vi "Sequencer Main - Copy.vi"() -> ()   [LabVIEW 2018] (continued)
                              n2084 = Add(1:w4034, 2:w4038) -> (0:w4062:dynamicdata)  [unwired: 1 in, 1 out]
                              n2085 = Multiply(x=w4027, y=w4022) -> (x*y=w4025:dynamicdata)
                              n2086 = Multiply(x=w4065, y=w4022) -> (x*y=w4061:dynamicdata)
                              n2087 = Multiply(x=w4064, y=w4022) -> (x*y=w4060:dynamicdata)
                              n2088 = local read "Measure Ch-A"() -> (w4069:T10)
                              n2089 = Multiply(x=w4030, y=w4022) -> (x*y=w4024:dynamicdata)
                              n2090 = Multiply(x=w4063, y=w4022) -> (x*y=w4059:dynamicdata)
                              n2091 = Multiply(x=w4062, y=w4022) -> (x*y=w4058:dynamicdata)
                              n2092 = Bundle By Name(cluster=w4069, "MAX Vpp"=w4061, "PickToPoick / 2"=w4025, "MIN Vpp"=w4060) -> (w4068:T10)
                              n2093 = local read "Measure Ch-B"() -> (w4066:T9)
                              n2094 = Bundle By Name(cluster=w4066, "MAX Vpp"=w4059, "PickToPick / 2"=w4024, "MIN Vpp"=w4058) -> (w4067:T9)
                              n2095 = local write "Measure Ch-B"(w4067) -> ()
                              n2096 = local write "Measure Ch-A"(w4068) -> ()
                            }
                            frame #2 {
                              # "GoTo Test-nmb"
                              # "ReTest Cyckles"
                              # "Select Channel & Set Retest Parametrs in FALSE Case"
                              n2097 = Index Array(array=w4082, index #1=0 ("index"), index #2=1 ("index"), index #3=2 ("index")) -> (element #1=w4086:string, element #2=w4087:string, element #3=w4088:string)
                              n2098 = global read "Global Variable.vi" "Retest Cnt"() -> (w4081:i16)
                              n2099 = local read "Debugging"() -> (w4079:bool)
                              n2100 = To Upper Case(1:w4086) -> (0:w4078:string)
                              n2101 = call "Convert from Dynamic Data8"("Dynamic Data Type"=w4074) -> ("Scalar"=w4070:dbl)  [unwired: 3 in]
                              n2102 = call "Convert from Dynamic Data6"("Dynamic Data Type"=w4073) -> ("Scalar"=w4071:dbl)  [unwired: 3 in]
                              n2103 = Decimal String To Number(string=w4088) -> (number=w4075:i32)  [unwired: 2 in, 1 out]
                              n2104 = Decimal String To Number(string=w4087) -> (number=w4077:i32)  [unwired: 2 in, 1 out]
                              n2105 = Equal?(x=w4081, y=i16 0) -> (x = y?=w4076:bool)
                              n2106 = case shown="False" w4079 {
                                tunnel: w4078 -> [w4093 _]
                                tunnel: w4076 -> [w4090 _]
                                tunnel: w4075 -> [w4092 _]
                                tunnel: w4077 -> [w4091 _]
                                frame False {
                                n2107 = case shown="\"FALSE\"" w4093 {
                                tunnel: w4090 -> [_ w4097]
                                tunnel: w4092 -> [_ w4094]
                                tunnel: w4091 -> [_ w4095]
                                frame "Idle", Default {
                                }
                                frame "FALSE" {
                                n2108 = global write "Global Variable.vi" "Retest Step Nmb"(w4095) -> ()
                                n2109 = global write "Global Variable.vi" "Retest Nmb"(w4094) -> ()
                                n2110 = case shown="True" w4097 {
                                tunnel: w4094 -> [_ w4101]
                                tunnel: w4095 -> [_ _]
                                frame False {
                                n2111 = global read "Global Variable.vi" "Retest Cnt"() -> (w4099:i16)
                                n2112 = Decrement(x=w4099) -> (x-1=w4098:i16)
                                n2113 = global write "Global Variable.vi" "Retest Cnt"(w4098) -> ()
                                }
                                frame True {
                                # "if(Retest-OFF & Cnt=0)"
                                n2114 = Decrement(x=w4101) -> (x-1=w4100:i32)
                                n2115 = global write "Global Variable.vi" "Retest Cnt"(w4100) -> ()
                                }
                                }
                                n2116 = global write "Global Variable.vi" "Retest ON"(TRUE ("Retest ON")) -> ()
                                }
                                }
                                }
                                frame True {
                                }
                              }
                              n2117 = case shown="\"A\", Default" w4089 {
                                tunnel: [w4102 w4103] -> w4072
                                tunnel: w4071 -> [_ w4103]
                                tunnel: w4070 -> [w4102 _]
                                frame "A", Default {
                                }
                                frame "B" {
                                }
                              }
                            }
                            frame #3 {
                              n2118 = local read "Delay"() -> (w4104:u16)
                              n2119 = Multiply(x=w4104, y=u32 1000 ("milliseconds to wait")) -> (x*y=w4106:u32)
                              n2120 = Wait (ms)(milliseconds to wait=w4106) -> ()  [unwired: 1 out]
                            }
                          }
                          n2121 = in-place {
                            in-place-border: w3964 -> [w3987]
                            in-place-border: w3965 -> [w3981]
                            in-place-border: w3966 -> [w3980]
                            in-place-border: [w3988] -> w3962
                            in-place-border: [w3986] -> w3961
                            # "Step Result Msg"
                            # "Step TEST Result"
                            n2122 = In Range and Coerce(upper limit=w3981, x=w3987, lower limit=w3980) -> (In Range?=w3984:bool)  [unwired: 1 out]
                            n2123 = And(x=w3984, y=TRUE) -> (x .and. y?=w3983:bool)
                            n2124 = case shown="False" w3983 {
                              tunnel: [enum16{"Idle", "PASS", "FALSE"}."FALSE" ("Step Test Result") enum16{"Idle", "PASS", "FALSE"}."PASS" ("Step Test Result")] -> w3988
                              frame False {
                              }
                              frame True {
                              }
                            }
                            n2125 = Format Into String(format string="%.1f (V)", w3987) -> (resulting string=w3986:string)  [unwired: 2 in, 1 out]
                          }
                        }
                        frame 53 {
                          # "Read Only POSITIVE or NEGATIVE Values"
                          # "Read Arrays Of DATA"
                          # "Lover Lim"
                          # "Upper Lim"
                          # "PicoScope Case\nPositive / Negative"
                          # "PicoScope Case"
                          n2126 = Unbundle By Name(w4131) -> ("Parameters"=w4125:string, "Test Values.Upper Limit"=w4129:dbl, "Test Values.Lower Limit"=w4128:dbl, "Test Values.Numeric Value"=w4130:dbl)
                          n2127 = property on="Tab Control Msg" class="TabCtl (strict)"("Value"=T21."Scope" ("Tab Control Msg")) -> (error out=w4127:errorcluster)  [unwired: 2 in, 1 out]
                          n2128 = flat-sequence {
                            tunnel: w4130 -> [w4163]
                            tunnel: w4129 -> [w4156]
                            tunnel: w4128 -> [w4155]
                            tunnel: w4127 -> [_]
                            tunnel: [w4156] -> w4115
                            tunnel: [w4155] -> w4116
                            tunnel: w4125 -> [w4154]
                            tunnel: [w4152] -> w4120
                            tunnel: [w4149] -> w4117
                            tunnel: [w4146] -> w4109
                            tunnel: [w4194] -> w4124
                            tunnel: [w4193] -> w4123
                            tunnel: [w4192] -> w4122
                            tunnel: [w4191] -> w4121
                            tunnel: w4120 -> [w4180]
                            tunnel: [w4180] -> w4119
                            tunnel: [w4179] -> w4118
                            tunnel: w4117 -> [w4179]
                            tunnel: [w4177] -> w4110
                            tunnel: w4109 -> [w4177]
                            tunnel: [w4234] -> w4114
                            tunnel: [w4236] -> w4113
                            tunnel: w4124 -> [w4235]
                            tunnel: w4123 -> [w4233]
                            tunnel: w4122 -> [w4232]
                            tunnel: w4121 -> [w4231]
                            tunnel: w4119 -> [w4230]
                            tunnel: w4118 -> [w4223]
                            tunnel: w4110 -> [w4215]
                            tunnel: [w4214] -> w4108
                            frame #0 {
                              n2129 = while {
                                shift-right: [w4174] -> _
                                shift-left: w4154 -> [w4175]
                                tunnel: [w4171] -> w4153 mode=indexing
                                stop <- w4173 stop-if-true
                                # "Get Array of Parametrs"
                                n2130 = Match Pattern(string=w4175, regular expression=">") -> (before substring=w4171:string, after substring=w4174:string, offset past match=w4172:i32)  [unwired: 1 in, 1 out]
                                n2131 = Less Than 0?(x=w4172) -> (x < 0?=w4173:bool)
                              }
                              n2132 = Multiply(x=w4155, y=-0.2) -> (x*y=w4158:dbl)
                              n2133 = Bundle("Lower Limit"=w4155, "Upper Limit"=w4156, "Numeric Value"=w4163) -> (w4164:T36)  [unwired: 1 in]
                              n2134 = Multiply(x=w4156, y=0.2) -> (x*y=w4160:dbl)
                              n2135 = Add(x=w4158, y=w4155) -> (x+y=w4157:dbl)
                              n2136 = property on="Limits" class="Slide (strict)"("Value"=w4164) -> ()  [unwired: 2 in, 2 out]
                              n2137 = Add(x=w4160, y=w4156) -> (x+y=w4159:dbl)
                              n2138 = property on="Limits" class="Slide (strict)"("Scale.Maximum"=w4159, "Scale.Minimum"=w4157) -> ()  [unwired: 2 in, 2 out]
                              n2139 = Index Array(array=w4153, index #1=0 ("index"), index #2=1 ("index"), index #3=2 ("index")) -> (element #1=w4152:string, element #2=w4146:string, element #3=w4147:string)
                              n2140 = while {
                                shift-right: [w4168] -> _
                                shift-left: w4147 -> [w4169]
                                tunnel: [w4165] -> w4149 mode=indexing
                                stop <- w4167 stop-if-true
                                # "Get Array of Sub Parametrs"
                                n2141 = Match Pattern(string=w4169, regular expression=":") -> (before substring=w4165:string, after substring=w4168:string, offset past match=w4166:i32)  [unwired: 1 in, 1 out]
                                n2142 = Less Than 0?(x=w4166) -> (x < 0?=w4167:bool)
                              }
                            }
                            frame #1 {
                              w4184 = 700 ("index")
                              w4178 = 290.0
                              # "302"
                              # "Devider compensite"
                              # "remove first\nxx element (noise)"
                              # "Ch-B Negative Vmin"
                              # "Ch-B Positive Vmax"
                              # "Ch-A Negative Vmin"
                              # "Ch-A Positive Vmax"
                              # "Res Devider Compens\n100K / 10K"
                              # "Calculate Values"
                              n2143 = local read "Channel A"() -> (w4213:cluster{i32, dbl, dbl[]})
                              n2144 = local read "Channel B"() -> (w4208:cluster{i32, dbl, dbl[]})
                              n2145 = Unbundle(w4213) -> (w4181:dbl[])  [unwired: 2 out]
                              n2146 = Unbundle(w4208) -> (w4186:dbl[])  [unwired: 2 out]
                              n2147 = Array Size(array=w4181) -> (size(s)=w4189:i32)
                              n2148 = Array Size(array=w4186) -> (size(s)=w4185:i32)
                              n2149 = Subtract(x=w4189, y=w4184) -> (x-y=w4188:i32)
                              n2150 = Array Subset(array=w4181, index=w4184, length=w4188) -> (w4190:dbl[])
                              n2151 = Subtract(x=w4185, y=w4184) -> (x-y=w4183:i32)
                              n2152 = Array Subset(array=w4186, index=w4184, length=w4183) -> (w4187:dbl[])
                              n2153 = call-poly <vilib>:"Basic Averaged DC-RMS.vi"("signal in"=w4190) -> ("RMS value"=w4202:dbl, "DC value"=w4182:dbl)  [unwired: 7 in, 2 out]
                              n2154 = Array Max & Min(array=w4190) -> (max value=w4210:dbl, min value=w4209:dbl)  [unwired: 2 out]
                              n2155 = call-poly <vilib>:"Basic Averaged DC-RMS.vi"("signal in"=w4187) -> ("RMS value"=w4198:dbl, "DC value"=w4207:dbl)  [unwired: 7 in, 2 out]
                              n2156 = Array Max & Min(array=w4187) -> (max value=w4205:dbl, min value=w4206:dbl)  [unwired: 2 out]
                              n2157 = Subtract(x=w4210, y=w4182) -> (x-y=w4201:dbl)
                              n2158 = Add(x=w4209, y=w4182) -> (x+y=w4200:dbl)
                              n2159 = Subtract(x=w4205, y=w4207) -> (x-y=w4196:dbl)
                              n2160 = Add(x=w4206, y=w4207) -> (x+y=w4195:dbl)
                              n2161 = Multiply(x=w4202, y=w4178) -> (x*y=w4199:dbl)
                              n2162 = Multiply(x=w4201, y=w4178) -> (x*y=w4194:dbl)
                              n2163 = Multiply(x=w4200, y=w4178) -> (x*y=w4193:dbl)
                              n2164 = Multiply(x=w4198, y=w4178) -> (x*y=w4197:dbl)
                              n2165 = Multiply(x=w4196, y=w4178) -> (x*y=w4192:dbl)
                              n2166 = Multiply(x=w4195, y=w4178) -> (x*y=w4191:dbl)
                              n2167 = local read "Measure Ch-A"() -> (w4212:T10)
                              n2168 = Bundle By Name(cluster=w4212, "MAX Vpp"=w4194, "PickToPoick / 2"=w4199, "MIN Vpp"=w4193) -> (w4211:T10)
                              n2169 = local read "Measure Ch-B"() -> (w4203:T9)
                              n2170 = local write "Measure Ch-A"(w4211) -> ()
                              n2171 = Bundle By Name(cluster=w4203, "MAX Vpp"=w4192, "PickToPick / 2"=w4197, "MIN Vpp"=w4191) -> (w4204:T9)
                              n2172 = local write "Measure Ch-B"(w4204) -> ()
                            }
                            frame #2 {
                              # "Negative"
                              # "Positive"
                              # "GoTo Test-nmb"
                              # "ReTest Cyckles"
                              # "Select Channel & Set Retest Parametrs in FALSE Case"
                              n2173 = Index Array(array=w4223, index #1=0 ("index"), index #2=1 ("index"), index #3=2 ("index")) -> (element #1=w4227:string, element #2=w4228:string, element #3=w4229:string)
                              n2174 = global read "Global Variable.vi" "Retest Cnt"() -> (w4222:i16)
                              n2175 = local read "Debugging"() -> (w4220:bool)
                              n2176 = To Upper Case(1:w4227) -> (0:w4219:string)
                              n2177 = Decimal String To Number(string=w4229) -> (number=w4216:i32)  [unwired: 2 in, 1 out]
                              n2178 = Decimal String To Number(string=w4228) -> (number=w4218:i32)  [unwired: 2 in, 1 out]
                              n2179 = Equal?(x=w4222, y=i16 0) -> (x = y?=w4217:bool)
                              n2180 = case shown="False" w4220 {
                                tunnel: w4219 -> [w4240 _]
                                tunnel: w4217 -> [w4237 _]
                                tunnel: w4216 -> [w4239 _]
                                tunnel: w4218 -> [w4238 _]
                                frame False {
                                n2181 = case shown="\"FALSE\"" w4240 {
                                tunnel: w4237 -> [_ w4244]
                                tunnel: w4239 -> [_ w4241]
                                tunnel: w4238 -> [_ w4242]
                                frame "Idle", Default {
                                }
                                frame "FALSE" {
                                n2182 = global write "Global Variable.vi" "Retest Step Nmb"(w4242) -> ()
                                n2183 = global write "Global Variable.vi" "Retest Nmb"(w4241) -> ()
                                n2184 = case shown="True" w4244 {
                                tunnel: w4241 -> [_ w4248]
                                tunnel: w4242 -> [_ _]
                                frame False {
                                n2185 = global read "Global Variable.vi" "Retest Cnt"() -> (w4246:i16)
                                n2186 = Decrement(x=w4246) -> (x-1=w4245:i16)
                                n2187 = global write "Global Variable.vi" "Retest Cnt"(w4245) -> ()
                                }
                                frame True {
                                # "if(Retest-OFF & Cnt=0)"
                                n2188 = Decrement(x=w4248) -> (x-1=w4247:i32)
                                n2189 = global write "Global Variable.vi" "Retest Cnt"(w4247) -> ()
                                }
                                }
                                n2190 = global write "Global Variable.vi" "Retest ON"(TRUE ("Retest ON")) -> ()
                                }
                                }
                                }
                                frame True {
                                }
                              }
                              n2191 = case shown="\"A\", Default" w4230 {
                                tunnel: [w4250 w4252] -> w4236
                                tunnel: w4235 -> [w4250 _]
                                tunnel: [w4249 w4251] -> w4234
                                tunnel: w4233 -> [w4249 _]
                                tunnel: w4232 -> [_ w4252]
                                tunnel: w4231 -> [_ w4251]
                                frame "A", Default {
                                }
                                frame "B" {
                                }
                              }
                              n2192 = To Lower Case(string=w4215) -> (all lower case string=w4214:string)
                            }
                          }
                          n2193 = in-place {
                            in-place-border: w4113 -> [w4134]
                            in-place-border: w4114 -> [w4133]
                            in-place-border: w4115 -> [w4137]
                            in-place-border: w4116 -> [w4136]
                            in-place-border: [w4141] -> w4112
                            in-place-border: [w4140] -> w4111
                            in-place-border: w4108 -> [w4135]
                            # "Upper Limit Check"
                            # "Step Result Msg"
                            # "Step TEST Result"
                            n2194 = case shown="\"positive\", Default" w4135 {
                              tunnel: w4134 -> [_ w4143]
                              tunnel: w4133 -> [w4142 _]
                              tunnel: [w4142 w4143] -> w4132
                              frame "negative" {
                              }
                              frame "positive", Default {
                              }
                            }
                            n2195 = Format Into String(format string="%.1f (VAC )", w4132) -> (resulting string=w4140:string)  [unwired: 2 in, 1 out]
                            n2196 = In Range and Coerce(upper limit=w4137, x=w4132, lower limit=w4136) -> (In Range?=w4138:bool)  [unwired: 1 out]
                            n2197 = case shown="False" w4138 {
                              tunnel: [enum16{"Idle", "PASS", "FALSE"}."FALSE" ("Step Test Result") enum16{"Idle", "PASS", "FALSE"}."PASS" ("Step Test Result")] -> w4141
                              frame False {
                              }
                              frame True {
                              }
                            }
                          }
                        }
                        frame 54 {
                          # "PicoScope\n     Case\nLower Limit"
                          # "Read Arrays Of DATA"
                          # "Lover Lim"
                          # "Upper Lim"
                          # "PicoScope Case"
                          n2198 = Unbundle By Name(w4273) -> ("Parameters"=w4265:string, "Test Values.Upper Limit"=w4271:dbl, "Test Values.Lower Limit"=w4270:dbl, "Test Values.Numeric Value"=w4272:dbl)
                          n2199 = property on="Tab Control Msg" class="TabCtl (strict)"("Value"=T21."Scope" ("Tab Control Msg")) -> (error out=w4269:errorcluster)  [unwired: 2 in, 1 out]
                          n2200 = flat-sequence {
                            tunnel: w4272 -> [w4298]
                            tunnel: w4271 -> [w4291]
                            tunnel: w4270 -> [w4290]
                            tunnel: w4269 -> [_]
                            tunnel: [w4291] -> w4255
                            tunnel: [w4290] -> w4256
                            tunnel: w4265 -> [w4289]
                            tunnel: [w4287] -> w4260
                            tunnel: [w4283] -> w4257
                            tunnel: [w4328] -> w4264
                            tunnel: [w4327] -> w4263
                            tunnel: [w4326] -> w4262
                            tunnel: [w4325] -> w4261
                            tunnel: w4260 -> [w4314]
                            tunnel: [w4314] -> w4259
                            tunnel: [w4313] -> w4258
                            tunnel: w4257 -> [w4313]
                            tunnel: [w4366] -> w4254
                            tunnel: [w4368] -> w4253
                            tunnel: w4264 -> [w4367]
                            tunnel: w4263 -> [w4365]
                            tunnel: w4262 -> [w4364]
                            tunnel: w4261 -> [w4363]
                            tunnel: w4259 -> [w4362]
                            tunnel: w4258 -> [w4355]
                            frame #0 {
                              n2201 = while {
                                shift-right: [w4309] -> _
                                shift-left: w4289 -> [w4310]
                                tunnel: [w4306] -> w4288 mode=indexing
                                stop <- w4308 stop-if-true
                                # "Get Array of Parametrs"
                                n2202 = Match Pattern(string=w4310, regular expression=">") -> (before substring=w4306:string, after substring=w4309:string, offset past match=w4307:i32)  [unwired: 1 in, 1 out]
                                n2203 = Less Than 0?(x=w4307) -> (x < 0?=w4308:bool)
                              }
                              n2204 = Multiply(x=w4290, y=-0.2) -> (x*y=w4293:dbl)
                              n2205 = Bundle("Lower Limit"=w4290, "Upper Limit"=w4291, "Numeric Value"=w4298) -> (w4299:T36)  [unwired: 1 in]
                              n2206 = Multiply(x=w4291, y=0.2) -> (x*y=w4295:dbl)
                              n2207 = Add(x=w4293, y=w4290) -> (x+y=w4292:dbl)
                              n2208 = property on="Limits" class="Slide (strict)"("Value"=w4299) -> ()  [unwired: 2 in, 2 out]
                              n2209 = Add(x=w4295, y=w4291) -> (x+y=w4294:dbl)
                              n2210 = property on="Limits" class="Slide (strict)"("Scale.Maximum"=w4294, "Scale.Minimum"=w4292) -> ()  [unwired: 2 in, 2 out]
                              n2211 = Index Array(array=w4288, index #1=0 ("index"), index #2=1 ("index")) -> (element #1=w4287:string, element #2=w4284:string)
                              n2212 = while {
                                shift-right: [w4303] -> _
                                shift-left: w4284 -> [w4304]
                                tunnel: [w4300] -> w4283 mode=indexing
                                stop <- w4302 stop-if-true
                                # "Get Array of Sub Parametrs"
                                n2213 = Match Pattern(string=w4304, regular expression=":") -> (before substring=w4300:string, after substring=w4303:string, offset past match=w4301:i32)  [unwired: 1 in, 1 out]
                                n2214 = Less Than 0?(x=w4301) -> (x < 0?=w4302:bool)
                              }
                            }
                            frame #1 {
                              w4318 = 700 ("index")
                              w4312 = 290.0
                              # "302"
                              # "Devider compensite"
                              # "remove first\nxx element (noise)"
                              # "Ch-B Negative Vmin"
                              # "Ch-B Positive Vmax"
                              # "Ch-A Negative Vmin"
                              # "Ch-A Positive Vmax"
                              # "Res Devider Compens\n100K / 10K"
                              # "Calculate Values"
                              n2215 = local read "Channel A"() -> (w4347:cluster{i32, dbl, dbl[]})
                              n2216 = local read "Channel B"() -> (w4342:cluster{i32, dbl, dbl[]})
                              n2217 = Unbundle(w4347) -> (w4315:dbl[])  [unwired: 2 out]
                              n2218 = Unbundle(w4342) -> (w4320:dbl[])  [unwired: 2 out]
                              n2219 = Array Size(array=w4315) -> (size(s)=w4323:i32)
                              n2220 = Array Size(array=w4320) -> (size(s)=w4319:i32)
                              n2221 = Subtract(x=w4323, y=w4318) -> (x-y=w4322:i32)
                              n2222 = Array Subset(array=w4315, index=w4318, length=w4322) -> (w4324:dbl[])
                              n2223 = Subtract(x=w4319, y=w4318) -> (x-y=w4317:i32)
                              n2224 = Array Subset(array=w4320, index=w4318, length=w4317) -> (w4321:dbl[])
                              n2225 = call-poly <vilib>:"Basic Averaged DC-RMS.vi"("signal in"=w4324) -> ("RMS value"=w4336:dbl, "DC value"=w4316:dbl)  [unwired: 7 in, 2 out]
                              n2226 = Array Max & Min(array=w4324) -> (max value=w4344:dbl, min value=w4343:dbl)  [unwired: 2 out]
                              n2227 = call-poly <vilib>:"Basic Averaged DC-RMS.vi"("signal in"=w4321) -> ("RMS value"=w4332:dbl, "DC value"=w4341:dbl)  [unwired: 7 in, 2 out]
                              n2228 = Array Max & Min(array=w4321) -> (max value=w4339:dbl, min value=w4340:dbl)  [unwired: 2 out]
                              n2229 = Subtract(x=w4344, y=w4316) -> (x-y=w4335:dbl)
                              n2230 = Add(x=w4343, y=w4316) -> (x+y=w4334:dbl)
                              n2231 = Subtract(x=w4339, y=w4341) -> (x-y=w4330:dbl)
                              n2232 = Add(x=w4340, y=w4341) -> (x+y=w4329:dbl)
                              n2233 = Multiply(x=w4336, y=w4312) -> (x*y=w4333:dbl)
                              n2234 = Multiply(x=w4335, y=w4312) -> (x*y=w4328:dbl)
                              n2235 = Multiply(x=w4334, y=w4312) -> (x*y=w4327:dbl)
                              n2236 = Multiply(x=w4332, y=w4312) -> (x*y=w4331:dbl)
                              n2237 = Multiply(x=w4330, y=w4312) -> (x*y=w4326:dbl)
                              n2238 = Multiply(x=w4329, y=w4312) -> (x*y=w4325:dbl)
                              n2239 = local read "Measure Ch-A"() -> (w4346:T10)
                              n2240 = Bundle By Name(cluster=w4346, "MAX Vpp"=w4328, "PickToPoick / 2"=w4333, "MIN Vpp"=w4327) -> (w4345:T10)
                              n2241 = local read "Measure Ch-B"() -> (w4337:T9)
                              n2242 = local write "Measure Ch-A"(w4345) -> ()
                              n2243 = Bundle By Name(cluster=w4337, "MAX Vpp"=w4326, "PickToPick / 2"=w4331, "MIN Vpp"=w4325) -> (w4338:T9)
                              n2244 = local write "Measure Ch-B"(w4338) -> ()
                            }
                            frame #2 {
                              # "GoTo Test-nmb"
                              # "ReTest Cyckles"
                              # "Select Channel & Set Retest Parametrs in FALSE Case"
                              n2245 = case shown="\"B\"" w4362 {
                                tunnel: [w4382 w4384] -> w4368
                                tunnel: w4367 -> [w4382 _]
                                tunnel: [w4381 w4383] -> w4366
                                tunnel: w4365 -> [w4381 _]
                                tunnel: w4364 -> [_ w4384]
                                tunnel: w4363 -> [_ w4383]
                                frame "A", Default {
                                }
                                frame "B" {
                                }
                              }
                              n2246 = Index Array(array=w4355, index #1=0 ("index"), index #2=1 ("index"), index #3=2 ("index")) -> (element #1=w4359:string, element #2=w4360:string, element #3=w4361:string)
                              n2247 = global read "Global Variable.vi" "Retest Cnt"() -> (w4354:i16)
                              n2248 = local read "Debugging"() -> (w4352:bool)
                              n2249 = To Upper Case(1:w4359) -> (0:w4351:string)
                              n2250 = Decimal String To Number(string=w4361) -> (number=w4348:i32)  [unwired: 2 in, 1 out]
                              n2251 = Decimal String To Number(string=w4360) -> (number=w4350:i32)  [unwired: 2 in, 1 out]
                              n2252 = Equal?(x=w4354, y=i16 0) -> (x = y?=w4349:bool)
                              n2253 = case shown="False" w4352 {
                                tunnel: w4351 -> [w4372 _]
                                tunnel: w4349 -> [w4369 _]
                                tunnel: w4348 -> [w4371 _]
                                tunnel: w4350 -> [w4370 _]
                                frame False {
                                n2254 = case shown="\"FALSE\"" w4372 {
                                tunnel: w4369 -> [_ w4376]
                                tunnel: w4371 -> [_ w4373]
                                tunnel: w4370 -> [_ w4374]
                                frame "Idle", Default {
                                }
                                frame "FALSE" {
                                n2255 = global write "Global Variable.vi" "Retest Step Nmb"(w4374) -> ()
                                n2256 = global write "Global Variable.vi" "Retest Nmb"(w4373) -> ()
                                n2257 = case shown="True" w4376 {
                                tunnel: w4373 -> [_ w4380]
                                tunnel: w4374 -> [_ _]
                                frame False {
                                n2258 = global read "Global Variable.vi" "Retest Cnt"() -> (w4378:i16)
                                n2259 = Decrement(x=w4378) -> (x-1=w4377:i16)
                                n2260 = global write "Global Variable.vi" "Retest Cnt"(w4377) -> ()
                                }
                                frame True {
                                # "if(Retest-OFF & Cnt=0)"
                                n2261 = Decrement(x=w4380) -> (x-1=w4379:i32)
                                n2262 = global write "Global Variable.vi" "Retest Cnt"(w4379) -> ()
                                }
                                }
                                n2263 = global write "Global Variable.vi" "Retest ON"(TRUE ("Retest ON")) -> ()
                                }
                                }
                                }
                                frame True {
                                }
                              }
                            }
                          }
                          n2264 = in-place {
                            in-place-border: w4253 -> [_]
                            in-place-border: w4254 -> [w4277]
                            in-place-border: w4255 -> [w4275]
                            in-place-border: w4256 -> [w4274]
                            in-place-border: [w4280] -> w4267
                            in-place-border: [w4279] -> w4266
                            # "Step Result Msg"
                            # "Step TEST Result"
                            n2265 = In Range and Coerce(upper limit=w4275, x=w4277, lower limit=w4274) -> (In Range?=w4276:bool)  [unwired: 1 out]
                            n2266 = case shown="False" w4276 {
                              tunnel: [enum16{"Idle", "PASS", "FALSE"}."FALSE" ("Step Test Result") enum16{"Idle", "PASS", "FALSE"}."PASS" ("Step Test Result")] -> w4280
                              frame False {
                              }
                              frame True {
                              }
                            }
                            n2267 = Format Into String(format string="%.1f (VAC)", w4277) -> (resulting string=w4279:string)  [unwired: 2 in, 1 out]
                          }
                        }
                        frame 55 {
                          # "PicoScope\n     Case\nLower Limit"
                          # "Read Arrays Of DATA"
                          # "PicoScope AWG"
                          n2268 = Unbundle By Name(w4402) -> ("Parameters"=w4396:string, "Test Values.Upper Limit"=w4400:dbl, "Test Values.Lower Limit"=w4399:dbl, "Test Values.Numeric Value"=w4401:dbl)
                          n2269 = property on="Tab Control Msg" class="TabCtl (strict)"("Value"=T21."Settings" ("Tab Control Msg")) -> (error out=w4398:errorcluster)  [unwired: 2 in, 1 out]
                          n2270 = flat-sequence {
                            tunnel: w4401 -> [w4426]
                            tunnel: w4400 -> [w4419]
                            tunnel: w4399 -> [w4418]
                            tunnel: w4398 -> [_]
                            tunnel: [w4419] -> _
                            tunnel: [w4418] -> _
                            tunnel: w4396 -> [w4417]
                            tunnel: [w4415] -> w4395
                            tunnel: [w4409] -> w4392
                            tunnel: [w4408] -> w4391
                            tunnel: [w4407] -> w4390
                            tunnel: [w4406] -> w4389
                            tunnel: [w4405] -> w4388
                            tunnel: w4395 -> [w4454]
                            tunnel: w4392 -> [w4453]
                            tunnel: w4391 -> [w4452]
                            tunnel: w4390 -> [w4451]
                            tunnel: w4389 -> [w4450]
                            tunnel: w4388 -> [w4449]
                            tunnel: [w4447] -> w4387
                            frame #0 {
                              n2271 = while {
                                shift-right: [w4433] -> _
                                shift-left: w4417 -> [w4434]
                                tunnel: [w4429] -> w4416 mode=indexing
                                tunnel: [w4428] -> w4405
                                i -> [w4428]
                                stop <- w4432 stop-if-true
                                # "Get Array of Parametrs"
                                n2272 = Match Pattern(string=w4434, regular expression=">") -> (before substring=w4430:string, after substring=w4433:string, offset past match=w4431:i32)  [unwired: 1 in, 1 out]
                                n2273 = Less Than 0?(x=w4431) -> (x < 0?=w4432:bool)
                                n2274 = To Lower Case(string=w4430) -> (all lower case string=w4429:string)
                              }
                              n2275 = Multiply(x=w4418, y=-0.2) -> (x*y=w4421:dbl)
                              n2276 = Bundle("Lower Limit"=w4418, "Upper Limit"=w4419, "Numeric Value"=w4426) -> (w4427:T36)  [unwired: 1 in]
                              n2277 = Multiply(x=w4419, y=0.2) -> (x*y=w4423:dbl)
                              n2278 = Add(x=w4421, y=w4418) -> (x+y=w4420:dbl)
                              n2279 = Add(x=w4423, y=w4419) -> (x+y=w4422:dbl)
                              n2280 = property on="Limits" class="Slide (strict)"("Value"=w4427) -> ()  [unwired: 2 in, 2 out]
                              n2281 = property on="Limits" class="Slide (strict)"("Scale.Maximum"=w4422, "Scale.Minimum"=w4420) -> ()  [unwired: 2 in, 2 out]
                              n2282 = Index Array(array=w4416, index #1=0 ("index"), index #2=1 ("index"), index #3=2 ("index"), index #4=3 ("index"), index #5=4 ("index")) -> (element #1=w4415:string, element #2=w4409:string, element #3=w4408:string, element #4=w4407:string, element #5=w4406:string)
                            }
                            frame #1 {
                              n2283 = Not Equal?(x=w4449, y=4) -> (x != y?=w4436:bool)
                              n2284 = case shown="\"on\"" w4454 {
                                tunnel: w4453 -> [_ w4474]
                                tunnel: w4452 -> [_ w4473]
                                tunnel: w4451 -> [_ w4472]
                                tunnel: w4450 -> [_ w4471]
                                tunnel: [10000.0 w4462] -> w4438
                                tunnel: [w4456 w4461] -> w4445
                                tunnel: [w4455 w4460] -> w4444
                                tunnel: [w4455 w4459] -> w4443
                                tunnel: w4436 -> [_ w4458]
                                frame "off", Default {
                                w4455 = 0
                                w4456 = i16 0 items=["Sine"=0, "Square"=1, "Triangle"=2, "Ramp Up"=3, "Ramp Down"=4, "DC"=8, "Arbitrary"=6] ("Wave Type")
                                }
                                frame "on" {
                                w4465 = 1000000
                                n2285 = case shown="True" w4458 {
                                frame False {
                                }
                                frame True {
                                n2286 = One Button Dialog(message="PICo Scoê parameters\nErr!") -> ()  [unwired: 1 in, 1 out]
                                }
                                }
                                n2287 = Scan From String(input string=w4473) -> (output 1=w4468:dbl)  [unwired: 4 in, 3 out]
                                n2288 = Scan From String(input string=w4472) -> (output 1=w4467:dbl)  [unwired: 4 in, 3 out]
                                n2289 = Scan From String(input string=w4471) -> (output 1=w4466:dbl)  [unwired: 4 in, 3 out]
                                n2290 = Multiply(x=w4467, y=w4465) -> (x*y=w4464:dbl)
                                n2291 = Multiply(x=w4466, y=w4465) -> (x*y=w4463:dbl)
                                n2292 = To Long Integer(number=w4464) -> (32bit integer=w4460:i32)
                                n2293 = To Long Integer(number=w4463) -> (32bit integer=w4459:i32)
                                n2294 = case shown="\"triangle\"" w4474 {
                                tunnel: [w4478 w4479 w4480 w4481] -> w4461
                                frame "sine", Default {
                                w4478 = i16 0 items=["Sine"=0, "Square"=1, "Triangle"=2, "Ramp Up"=3, "Ramp Down"=4, "DC"=8, "Arbitrary"=6] ("Wave Type")
                                }
                                frame "square" {
                                w4479 = i16 1 items=["Sine"=0, "Square"=1, "Triangle"=2, "Ramp Up"=3, "Ramp Down"=4, "DC"=8, "Arbitrary"=6] ("Wave Type")
                                }
                                frame "triangle" {
                                w4480 = i16 2 items=["Sine"=0, "Square"=1, "Triangle"=2, "Ramp Up"=3, "Ramp Down"=4, "DC"=8, "Arbitrary"=6] ("Wave Type")
                                }
                                frame "dc" {
                                w4481 = i16 8 items=["Sine"=0, "Square"=1, "Triangle"=2, "Ramp Up"=3, "Ramp Down"=4, "DC"=8, "Arbitrary"=6] ("Wave Type")
                                }
                                }
                                n2295 = Greater Or Equal?(x=w4468, y=50000.0) -> (x >= y?=w4469:bool)
                                n2296 = case shown="True" w4469 {
                                tunnel: [w4476 50000.0] -> w4462
                                tunnel: w4468 -> [w4476 _]
                                frame False {
                                }
                                frame True {
                                }
                                }
                                }
                              }
                              n2297 = Bundle By Name(cluster=T29 {"Peak-to-Peak Voltage (microvolts)"=1000000, "Offset Voltage (microvolts)"=0, "Wave Type"=0, "Sweep Type"=0, "Shots"=0, "Sweeps"=0, "Trigger Type"=0, "Trigger Source"=0, "Ext. Threshold (ADC count)"=0, "White Noise"=FALSE} ("General AWG Settings"), "Wave Type"=w4445, "Peak-to-Peak Voltage (microvolts)"=w4444, "Offset Voltage (microvolts)"=w4443) -> (w4442:T29)
                              n2298 = global read "Global Variable.vi" "PicoScope Handle"() -> (w4441:u32)
                              n2299 = Bundle By Name(cluster=T30 {"Start Frequency"=1000.0, "Stop Frequency"=1000.0, "Increment"=0.0, "Dwell Time (seconds)"=0.0} ("Standard Waveform Settings"), "Start Frequency"=w4438, "Stop Frequency"=w4438) -> (w4439:T30)
                              n2300 = call "PicoScope2000aAWG.vi"("Standard Waveform Settings"=w4439, "General AWG Settings"=w4442, "Handle In"=w4441) -> ("error out"=w4446:errorcluster)  [unwired: 5 in, 3 out]
                              n2301 = call "PicoErrorHandler.vi"("error in"=w4446) -> ("error out"=w4447:errorcluster)
                              n2302 = call <userlib>:"Clear All Errors__ogtk.vi"("Error In"=w4447) -> ()  [unwired: 3 in, 1 out]
                            }
                          }
                          n2303 = Unbundle By Name(w4387) -> ("status"=w4385:bool)
                          n2304 = Not(x=w4385) -> (.not. x?=w4386:bool)
                          n2305 = case shown="True" w4386 {
                            tunnel: [enum16{"Idle", "PASS", "FALSE"}."FALSE" ("Step Test Result") enum16{"Idle", "PASS", "FALSE"}."PASS" ("Step Test Result")] -> w4393
                            frame False {
                            }
                            frame True {
                            }
                          }
                        }
                        frame 60 {
                          w4498 = "------------------------" ("string")
                          w4497 = "\r\n"
                          # "Step TEST Result"
                          # "Step Result Msg"
                          # "Str with \"false\" goto parameters"
                          # "Str \"false\" Preset"
                          # "Cmd Case"
                          # "Cmd Case"
                          n2306 = Unbundle By Name(w4511) -> ("Parameters"=w4493:string, "Step Description"=w4482:string, "Test Values.Numeric Value"=w4487:dbl, "Test Values.Upper Limit"=w4486:dbl, "Test Values.Lower Limit"=w4485:dbl)
                          n2307 = in-place {
                            in-place-border: w4493 -> [w4543]
                            in-place-border: [w4542] -> w4492
                            in-place-border: [w4541] -> w4490
                            # "STr \"fase\" exist"
                            n2308 = To Lower Case(string=w4543) -> (all lower case string=w4544:string)
                            n2309 = Match Pattern(string=w4544, regular expression="false") -> (after substring=w4546:string, offset past match=w4547:i32)  [unwired: 1 in, 2 out]
                            n2310 = Greater Or Equal To 0?(x=w4547) -> (x >= 0?=w4541:bool)
                            n2311 = case shown="True" w4541 {
                              tunnel: w4546 -> [_ w4550]
                              tunnel: [string[] [] w4549] -> w4542
                              frame False {
                                (unwired) ""
                              }
                              frame True {
                                n2312 = while {
                                shift-right: [w4554] -> _
                                shift-left: w4550 -> [w4555]
                                tunnel: [w4551] -> w4549 mode=indexing
                                stop <- w4553 stop-if-true
                                # "Get Array of Sub Parametrs"
                                n2313 = Match Pattern(string=w4555, regular expression=":") -> (before substring=w4551:string, after substring=w4554:string, offset past match=w4552:i32)  [unwired: 1 in, 1 out]
                                n2314 = Less Than 0?(x=w4552) -> (x < 0?=w4553:bool)
                                }
                              }
                            }
                          }
                          n2315 = while {
                            shift-right: [w4560] -> _
                            shift-left: w4493 -> [w4561]
                            tunnel: [w4557] -> w4495 mode=indexing
                            stop <- w4559 stop-if-true
                            # "Get Array of Parametrs"
                            n2316 = Match Pattern(string=w4561, regular expression=">") -> (before substring=w4557:string, after substring=w4560:string, offset past match=w4558:i32)  [unwired: 1 in, 1 out]
                            n2317 = Less Than 0?(x=w4558) -> (x < 0?=w4559:bool)
                          }
                          n2318 = Concatenate Strings(w4482, w4497, w4498, w4498, w4498, w4497) -> (w4499:string)
                          n2319 = property on="Tab Control Msg" class="TabCtl (strict)"("Value"=T21."Serial" ("Tab Control Msg")) -> (error out=w4509:errorcluster)  [unwired: 2 in, 1 out]
                          n2320 = property on="Serial CMD Mon" class="Str"("Value"=w4499) -> ()  [unwired: 2 in, 2 out]
                          n2321 = Index Array(array=w4495, index=0) -> (element=w4507:string)
                          n2322 = Index Array(array=w4495, index=1) -> (element=w4505:string)
                          n2323 = Index Array(array=w4495, index=2) -> (element=w4502:string)
                          n2324 = Index Array(array=w4495, index=3) -> (element=w4500:string)
                          n2325 = Index Array(array=w4495, index=4) -> (element=w4494:string)
                          n2326 = case shown="\"readcputemp\"" w4507 {
                            tunnel: w4509 -> [_ _ _ _ _ _ _ _ _ _ _ _ _ _ _ _ _ _ _]
                            tunnel: [enum16{"Idle", "PASS", "FALSE"}."FALSE" ("Step Test Result") w4571 w4609 w4636 w4677 w4727 w4871 w4909 w4953 w5129 w5198 w5353 w5401 w5448 w5482 w5517 w5552 w5582 w5613] -> w4508
                            tunnel: w4505 -> [_ w4569 _ _ _ w4739 w4875 w4907 _ w5127 w5224 _ _ w5449 _ w5518 _ w5580 _]
                            tunnel: w4502 -> [_ _ _ _ _ w4738 w4874 _ _ w5115 w5223 _ _ _ _ _ _ _ _]
                            tunnel: w4500 -> [_ _ _ _ _ w4737 w4873 _ _ _ _ _ _ _ _ _ _ _ _]
                            tunnel: w4494 -> [_ _ _ _ _ w4736 w4872 _ _ _ _ _ _ _ _ _ _ _ _]
                            tunnel: ["" w4568 w4606 w4634 w4668 w4726 w4870 w4905 w4951 w5114 w5218 "Set capmem '1' then '0' " w5400 w5447 _ _ w5550 _ _] -> w4484
                            tunnel: w4487 -> [_ _ _ _ _ _ _ _ _ _ _ _ _ _ _ _ _ _ _]
                            tunnel: w4486 -> [_ _ _ _ _ _ _ _ _ _ _ _ w5407 _ _ _ _ _ _]
                            tunnel: w4485 -> [_ _ _ _ _ _ _ _ _ _ _ _ w5406 _ _ _ _ _ _]
                            tunnel: ["" w4567 w4608 w4633 w4667 w4725 w4869 w4904 w4950 w5106 w5197 w5351 w5398 w5446 w5481 w5516 w5549 w5579 w5612] -> w4483
                            frame "False", Default {
                              n2327 = One Button Dialog(message="!Sequencer File Err") -> ()  [unwired: 1 in, 1 out]
                            }
                            frame "open" {
                              # "Param"
                              # "Cmd"
                              n2328 = flat-sequence {
                                tunnel: [w4582] -> w4573
                                tunnel: [w4581] -> w4572
                                tunnel: [w4580] -> w4570
                                tunnel: w4573 -> [w4586]
                                tunnel: w4572 -> [w4588]
                                tunnel: [w4589] -> w4571
                                tunnel: w4570 -> [w4583]
                                tunnel: w4569 -> [w4587]
                                tunnel: [w4584] -> w4568
                                tunnel: [w4583] -> w4567
                                frame #0 {
                                n2329 = global read "Global Variable.vi" "COM Port FTDI RS232"() -> (w4579:refnum<visa-resource-name>)
                                n2330 = call "ADB-Serial_WrRd.vi"("Tx Deay"=u16 1, "Timeout(Sec)"=1.0, "PassString"="Chuck(1)", "Command"="open", "ComPort"=w4579) -> ("error out"=w4581:errorcluster, "PASS"=w4582:bool, "received"=w4580:string)  [unwired: 4 in]
                                n2331 = invoke on="Serial CMD Mon" class="Str" method="Append String"("string"=w4580) -> ()  [unwired: 3 in, 4 out]
                                n2332 = Wait (ms)(milliseconds to wait=u32 500) -> ()  [unwired: 1 out]
                                }
                                frame #1 {
                                n2333 = case shown="True" w4586 {
                                tunnel: w4583 -> [_ w4596]
                                tunnel: w4587 -> [_ w4602]
                                tunnel: [FALSE w4599] -> w4585
                                tunnel: ["!Firmware vertion not Right" ("line") w4595] -> w4584
                                frame False {
                                }
                                frame True {
                                n2334 = call <userlib>:"Multi-line String to Array__ogtk.vi"("string"=w4596) -> ("lines"=w4598:string[])
                                n2335 = To Lower Case(string=w4602) -> (all lower case string=w4601:string)
                                n2336 = To Lower Case(string=w4596) -> (all lower case string=w4603:string)
                                n2337 = Match Pattern(string=w4603, regular expression=w4601) -> (offset past match=w4600:i32)  [unwired: 1 in, 3 out]
                                n2338 = Index Array(array=w4598, index=2) -> (element=w4595:string)
                                n2339 = Greater Than 0?(x=w4600) -> (x > 0?=w4599:bool)
                                }
                                }
                                n2340 = global read "Global Variable.vi" "Array Errors"() -> (w4592:errorcluster[])
                                n2341 = Replace Array Subset(array=w4592, new element=w4588, index=3) -> (w4591:errorcluster[])
                                n2342 = global write "Global Variable.vi" "Array Errors"(w4591) -> ()
                                n2343 = case shown="True" w4585 {
                                tunnel: [enum16{"Idle", "PASS", "FALSE"}."FALSE" ("Step Test Result") enum16{"Idle", "PASS", "FALSE"}."PASS" ("Step Test Result")] -> w4589
                                frame False {
                                # "Step TEST Result"
                                }
                                frame True {
                                # "Step TEST Result"
                                }
                                }
                                }
                              }
                            }
                            frame "passwd" {
                              n2344 = flat-sequence {
                                tunnel: [w4620] -> w4611
                                tunnel: [w4619] -> w4610
                                tunnel: [w4618] -> w4607
                                tunnel: w4611 -> [w4623]
                                tunnel: w4610 -> [w4624]
                                tunnel: [w4625] -> w4609
                                tunnel: [w4622] -> w4608
                                tunnel: w4607 -> [w4622]
                                tunnel: [w4621] -> w4606
                                frame #0 {
                                n2345 = global read "Global Variable.vi" "COM Port FTDI RS232"() -> (w4617:refnum<visa-resource-name>)
                                n2346 = call "ADB-Serial_WrRd.vi"("Tx Deay"=u16 1, "Timeout(Sec)"=1.0, "PassString"="Chuck(3)", "Command"="passwd admin", "ComPort"=w4617) -> ("error out"=w4619:errorcluster, "PASS"=w4620:bool, "received"=w4618:string)  [unwired: 4 in]
                                n2347 = invoke on="Serial CMD Mon" class="Str" method="Append String"("string"=w4618) -> ()  [unwired: 3 in, 4 out]
                                n2348 = Wait (ms)(milliseconds to wait=u32 250) -> ()  [unwired: 1 out]
                                }
                                frame #1 {
                                n2349 = global read "Global Variable.vi" "Array Errors"() -> (w4628:errorcluster[])
                                n2350 = case shown="False" w4623 {
                                tunnel: [enum16{"Idle", "PASS", "FALSE"}."FALSE" ("Step Test Result") enum16{"Idle", "PASS", "FALSE"}."PASS" ("Step Test Result")] -> w4625
                                tunnel: ["Err" "Admin"] -> w4621
                                frame False {
                                # "Step TEST Result"
                                }
                                frame True {
                                # "Step TEST Result"
                                }
                                }
                                n2351 = Replace Array Subset(array=w4628, new element=w4624, index=3) -> (w4627:errorcluster[])
                                n2352 = global write "Global Variable.vi" "Array Errors"(w4627) -> ()
                                }
                              }
                            }
                            frame "getpid" {
                              # "Param"
                              # "Cmd"
                              n2353 = flat-sequence {
                                tunnel: [w4646] -> w4638
                                tunnel: [w4645] -> w4637
                                tunnel: [w4644] -> w4635
                                tunnel: [w4644] -> _
                                tunnel: [w4644] -> w4633
                                tunnel: w4638 -> [w4650]
                                tunnel: w4637 -> [w4653]
                                tunnel: [w4654] -> w4636
                                tunnel: [w4647] -> w4634
                                tunnel: w4635 -> [w4651]
